vi "syncAIandAOat1MHz_v2.vi"() -> ()   [LabVIEW 2015]
uses:
  <vilib>/DAQmx/write.llb/DAQmx Write (Analog 1D Wfm NChan NSamp).vi
  <vilib>/DAQmx/read.llb/DAQmx Read (Analog 2D I16 NChan NSamp).vi
  <vilib>/DAQmx/write.llb/DAQmx Write (Analog 2D DBL NChan NSamp).vi
  <vilib>/Waveform/DWDTOps.llb/DWDT Analog to Digital.vi
  <vilib>/DAQmx/create/channels.llb/DAQmx Create Channel (AO-Voltage-Basic).vi
  <vilib>/DAQmx/create/channels.llb/DAQmx Create Channel (AI-Voltage-Basic).vi
  <vilib>/DAQmx/configure/timing.llb/DAQmx Timing (Sample Clock).vi
  <vilib>/DAQmx/miscellaneous.llb/DAQmx Fill In Error Info.vi
  <vilib>/DAQmx/configure/trigger.llb/DAQmx Start Trigger (Digital Edge).vi
  <resource>/objmgr/daqmx.rc
panel:
  in  "index (page)":i32
  out "XY Graph":T1(graph)
  in  "V":dbl=2.0 format="%#_13g"
  in  "AOrate":dbl=400000.0 format="%#_13g"
  in  "stop":bool
  out "Intensity Graph":sgl[][](graph)
  in  "error in 2":errorcluster caption="error in"
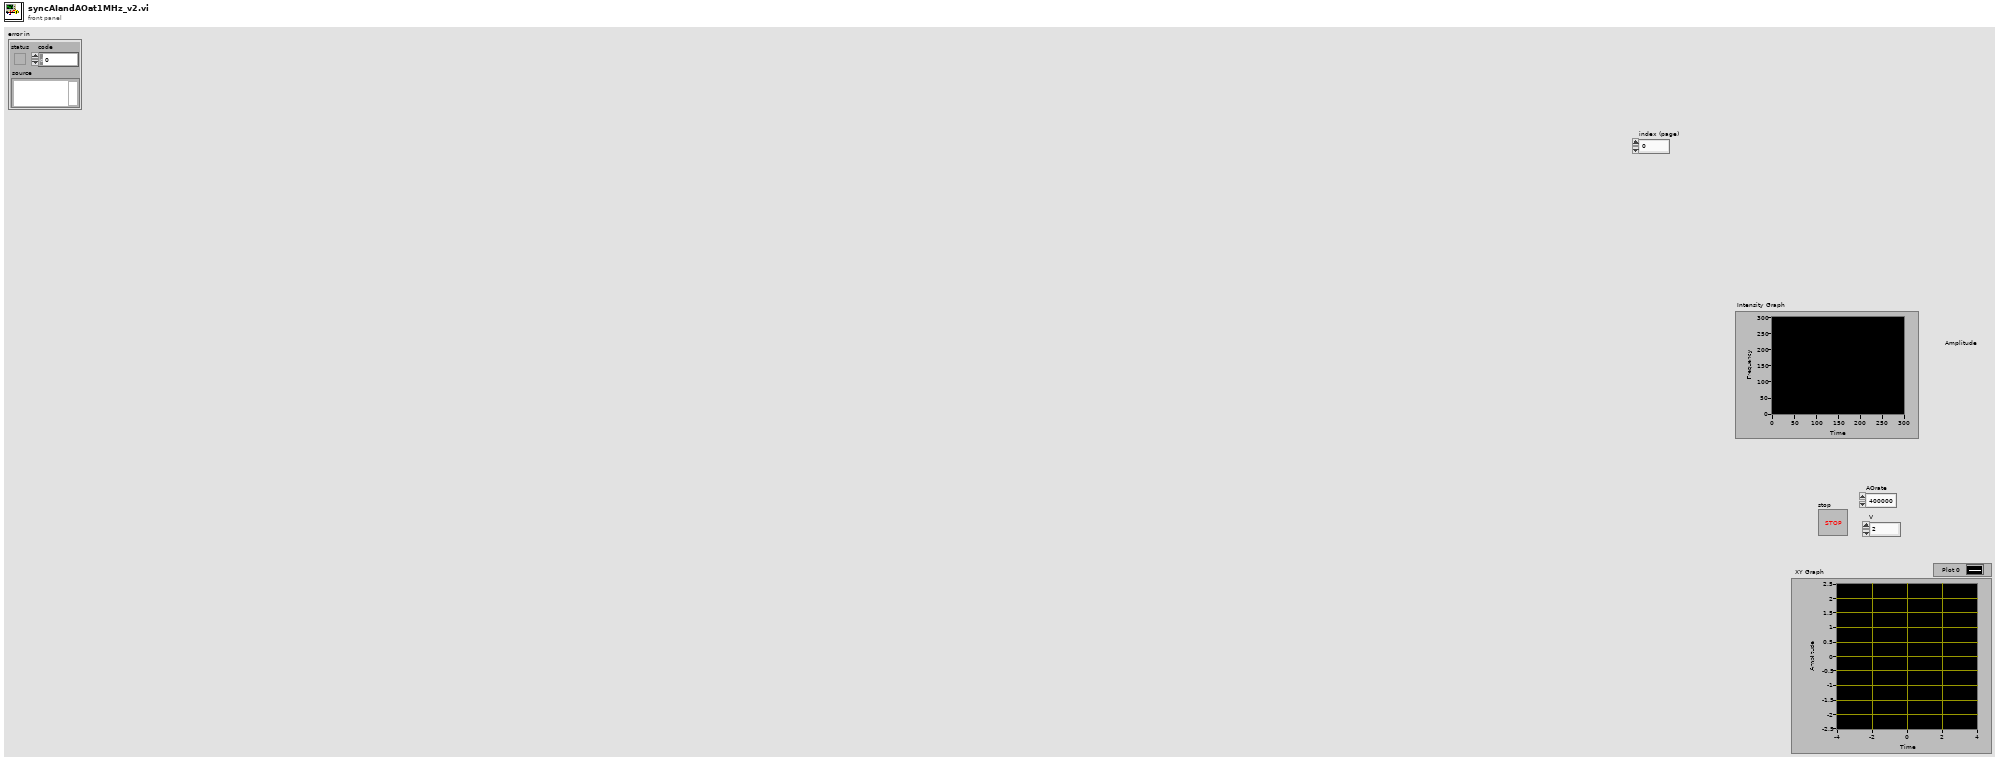
[diagram p1: front panel]
types:
  T1 = cluster{"X-WaveArray":dbl[], "Y-WaveArray":dbl[]}
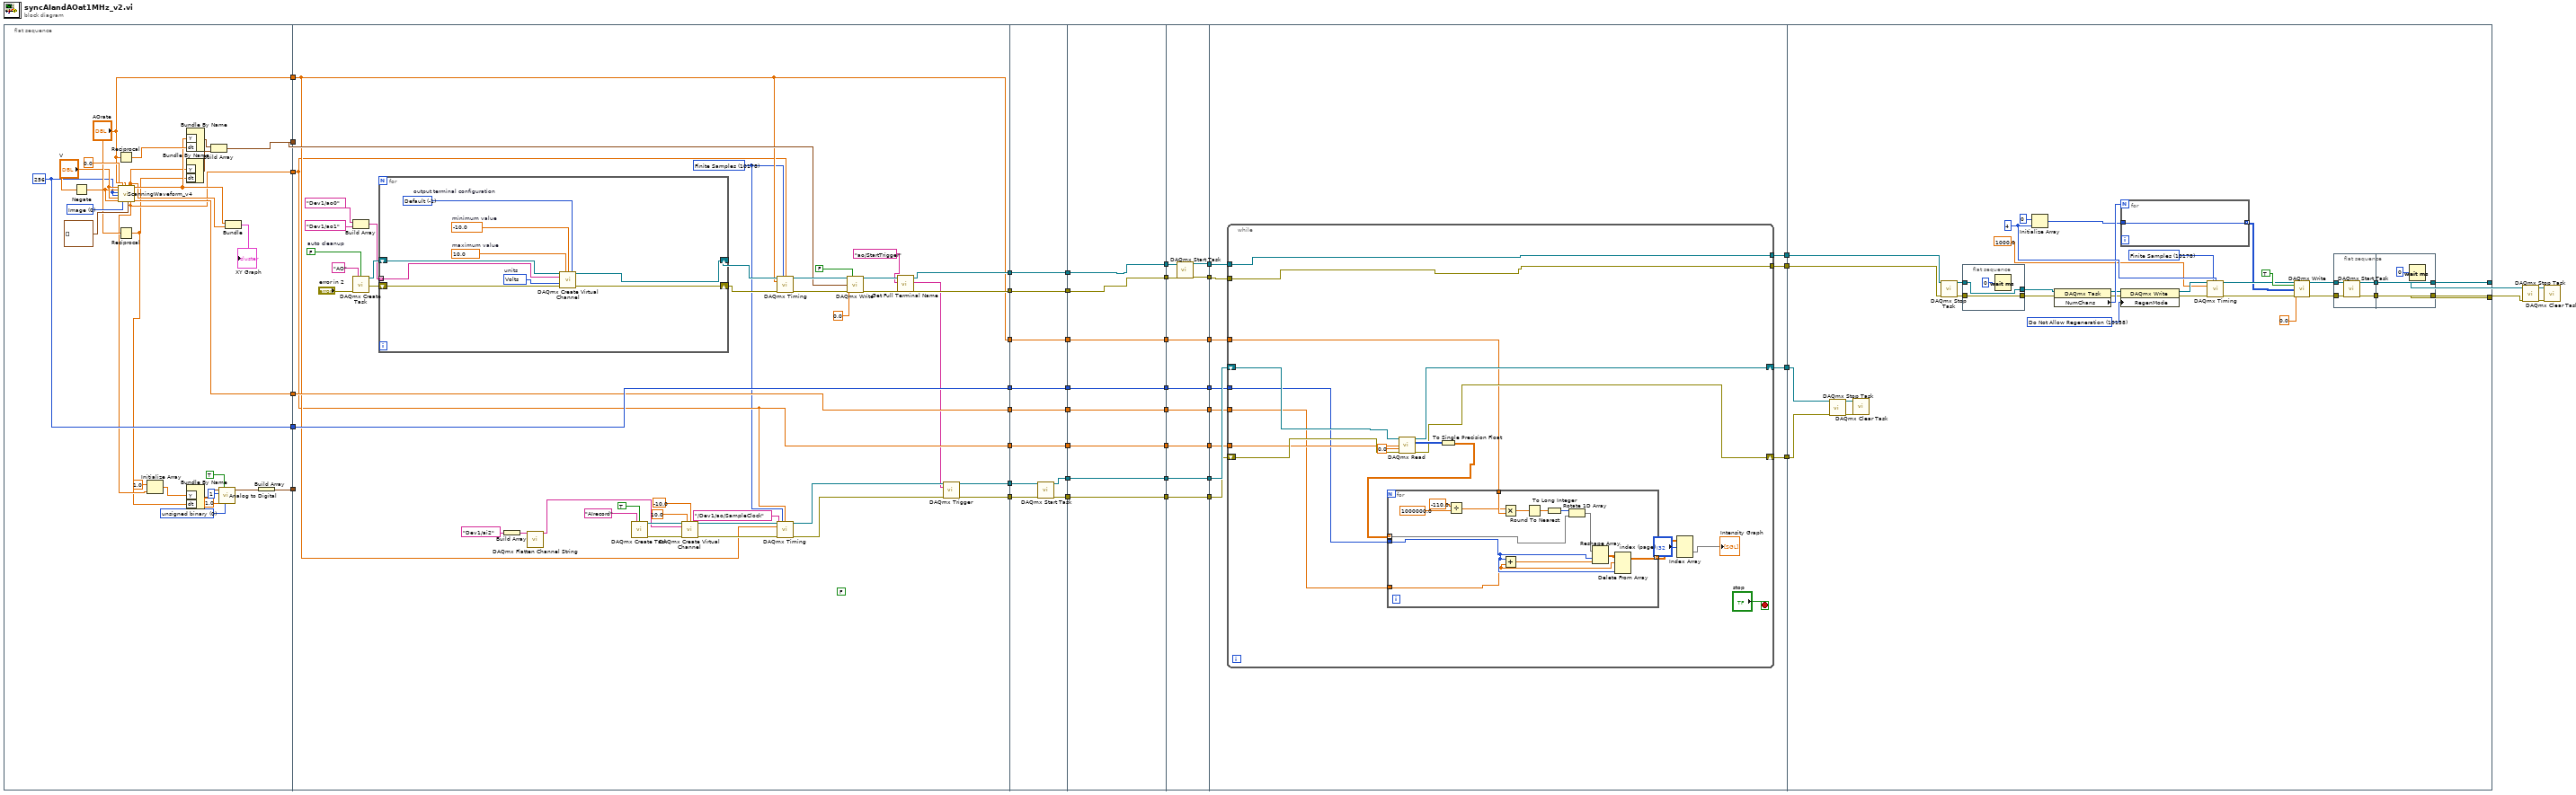
[diagram p0: block diagram]
diagram:
  n1 = flat-sequence {
    tunnel: [w61] -> w46
    tunnel: [w57] -> w45
    tunnel: ["AOrate"] -> w44
    tunnel: [w63] -> w20
    tunnel: [w62] -> w15
    tunnel: [w47] -> w7
    tunnel: w46 -> [w101]
    tunnel: w45 -> [w76]
    tunnel: w44 -> [w77]
    tunnel: [w83] -> w43
    tunnel: [w89] -> w40
    tunnel: [w87] -> w39
    tunnel: [w76] -> w25
    tunnel: [w77] -> w21
    tunnel: w20 -> [w91]
    tunnel: [w91] -> w16
    tunnel: w15 -> [w90]
    tunnel: [w90] -> w11
    tunnel: [w82] -> w10
    tunnel: w7 -> [_]
    tunnel: w43 -> [w133]
    tunnel: [w133] -> w42
    tunnel: [w132] -> w41
    tunnel: w40 -> [w131]
    tunnel: w39 -> [w130]
    tunnel: [w129] -> w33
    tunnel: [w128] -> w31
    tunnel: [w127] -> w26
    tunnel: w25 -> [w127]
    tunnel: [w126] -> w22
    tunnel: w21 -> [w126]
    tunnel: [w125] -> w17
    tunnel: w16 -> [w125]
    tunnel: [w124] -> w12
    tunnel: w11 -> [w124]
    tunnel: w10 -> [w132]
    tunnel: w42 -> [w135]
    tunnel: w41 -> [w134]
    tunnel: [w135] -> w38
    tunnel: [w134] -> w36
    tunnel: [w141] -> w34
    tunnel: w33 -> [w141]
    tunnel: [w140] -> w32
    tunnel: w31 -> [w140]
    tunnel: [w139] -> w27
    tunnel: w26 -> [w139]
    tunnel: [w138] -> w23
    tunnel: w22 -> [w138]
    tunnel: [w137] -> w18
    tunnel: w17 -> [w137]
    tunnel: [w136] -> w13
    tunnel: w12 -> [w136]
    tunnel: w38 -> [w145]
    tunnel: [w143] -> w37
    tunnel: w36 -> [w144]
    tunnel: [w142] -> w35
    tunnel: w34 -> [w151]
    tunnel: w32 -> [w150]
    tunnel: [w151] -> w30
    tunnel: [w150] -> w29
    tunnel: [w149] -> w28
    tunnel: w27 -> [w149]
    tunnel: [w148] -> w24
    tunnel: w23 -> [w148]
    tunnel: [w147] -> w19
    tunnel: w18 -> [w147]
    tunnel: [w146] -> w14
    tunnel: w13 -> [w146]
    tunnel: w37 -> [w154]
    tunnel: w35 -> [w155]
    tunnel: w30 -> [w163]
    tunnel: w29 -> [w162]
    tunnel: w28 -> [w161]
    tunnel: w24 -> [w158]
    tunnel: w19 -> [w157]
    tunnel: w14 -> [w156]
    tunnel: [w160] -> w4
    tunnel: [w159] -> w3
    tunnel: [w153] -> w2
    tunnel: [w152] -> w1
    tunnel: [w204] -> w6
    tunnel: [w203] -> w5
    tunnel: w1 -> [w205]
    tunnel: w2 -> [w206]
    tunnel: w3 -> [w199]
    tunnel: w4 -> [w200]
    frame #0 {
      w49 = u16 0 items=["unsigned binary", "offset binary", "2's complement"] ("data format (offset binary)")
      w63 = 256
      w71 = u16 0 items=["Image", "Fill Rectangle", "Fill Circle", "Draw Freeform", "Fill Freeform", "Ellipse Boundary", "Line"] ("Drawing Mode")
      n2 = Negate(x="V") -> (-x=w64:dbl)
      n3 = Reciprocal(x="AOrate") -> (1/x=w69:dbl)
      n4 = Reciprocal(x="AOrate") -> (1/x=w54:dbl)
      n5 = call "ScanningWaveform_v4.vi"("Vy-min"=w64, "Vy-max"="V", "yPixels/tPixels"=w63, "xPixels/rPixels"=w63, "Vx-min"=w64, "Vx-max"="V", "Drawing Mode"=w71, "Angle"=0.0, "AOrate"="AOrate", "Points"=cluster{"X":dbl, "Y":dbl}[] []) -> ("numPixels"=w57:dbl, "Y-WaveArray"=w59:dbl[], "P"=w62:dbl, "X-WaveArray"=w60:dbl[])  [unwired: 6 in]
      n6 = Initialize Array(1.0 ("element"), w57) -> (w55:dbl[])
      n7 = Bundle By Name("Y"=w59, "dt"=w54) -> (w67:waveform(dbl))  [unwired: 1 in]
      n8 = Bundle By Name("Y"=w60, "dt"=w69) -> (w68:waveform(dbl))  [unwired: 1 in]
      n9 = Bundle By Name("Y"=w55, "dt"=w54) -> (w53:waveform(dbl))  [unwired: 1 in]
      n10 = Build Array(w68, w67) -> (w61:waveform(dbl)[])
      n11 = call-poly <vilib>:"Analog to Digital.vi"("data format (offset binary)"=w49, "compress digital (T)"=TRUE, "full-scale range (pk-pk)"=1.0, "resolution (16 bit)"=1, "analog waveform"=w53) -> ("digital waveform"=w48:digitalwaveform)  [unwired: 3 in, 3 out]
      n12 = Bundle("X-WaveArray"=w60, "Y-WaveArray"=w59) -> (→"XY Graph":T1)  [unwired: 1 in]
      n13 = Build Array(w48) -> (w47:digitalwaveform[])
    }
    frame #1 {
      (unwired) FALSE ("auto start")
      w75 = 10178 items=["Finite Samples"=10178, "Continuous Samples"=10123, "Hardware Timed Single Point"=12522] ("sample mode")
      w112 = FALSE  # auto cleanup
      n14 = Build Array(tag "Dev1/ao0" ("physical channels"), tag "Dev1/ao1" ("physical channels")) -> (w102:tag[])
      n15 = call <vilib>:"DAQmx Create Task.vi"("new task name"="AO", "auto cleanup"=w112, "error in"="error in 2") -> ("task out"=w113:refnum<k21>, "error out"=w114:errorcluster)  [unwired: 11 in]
      n16 = for {
        shift-right: [w116] -> w109
        shift-left: w113 -> [w119]
        shift-right: [w115] -> w108
        shift-left: w114 -> [w118]
        tunnel: w102 -> [w117] mode=indexing
        w123 = -1 items=["Default"=-1, "RSE"=10083, "Differential"=10106, "Pseudodifferential"=12529]  # output terminal configuration
        w122 = 10348 items=["Volts"=10348, "From Custom Scale"=10065]  # units
        w121 = -10.0  # minimum value
        w120 = 10.0  # maximum value
        n17 = call-poly <vilib>:"DAQmx Create Virtual Channel.vi"("task in"=w119, "maximum value"=w120, "minimum value"=w121, "output terminal configuration"=w123, "physical channels"=w117, "units"=w122, "error in"=w118) -> ("task out"=w116:refnum<k21>, "error out"=w115:errorcluster)  [unwired: 7 in]
      }
      n18 = Build Array(tag "Dev1/ai2" ("physical channels")) -> (w80:tag[])
      n19 = call <vilib>:"DAQmx Flatten Channel String.vi"("names in"=w80) -> ("names out"=w78:string)  [unwired: 13 in, 1 out]
      n20 = call <vilib>:"DAQmx Create Task.vi"("new task name"="AIrecord", "auto cleanup"=TRUE) -> ("task out"=w94:refnum<k21>, "error out"=w95:errorcluster)  [unwired: 12 in]
      n21 = call-poly <vilib>:"DAQmx Create Virtual Channel.vi"("task in"=w94, "maximum value"=10.0, "minimum value"=-10.0, "physical channels"=w78, "error in"=w95) -> ("task out"=w100:refnum<k21>, "error out"=w99:errorcluster)  [unwired: 9 in]
      n22 = call-poly <vilib>:"DAQmx Timing.vi"("task/channels in"=w100, "sample mode"=w75, "samples per channel"=w76, "rate"=w77, "source"=tag "/Dev1/ao/SampleClock", "error in"=w99) -> ("task out"=w92:refnum<k21>, "error out"=w88:errorcluster)  [unwired: 8 in]
      n23 = call-poly <vilib>:"DAQmx Timing.vi"("task/channels in"=w109, "sample mode"=w75, "samples per channel"=w76, "rate"=w77, "error in"=w108) -> ("task out"=w107:refnum<k21>, "error out"=w106:errorcluster)  [unwired: 2 in, 7 out]
      n24 = call-poly <vilib>:"DAQmx Write.vi"("task/channels in"=w107, "auto start"=FALSE, "data"=w101, "timeout"=0.0, "error in"=w106) -> ("task out"=w86:refnum<k21>, "error out"=w85:errorcluster)  [unwired: 8 in, 1 out]
      n25 = call "Get Full Terminal Name.vi"("error in"=w85, "Local Terminal Name"="ao/StartTrigger", "task/channels in"=w86) -> ("error out"=w82:errorcluster, "Terminal Name with Device Prefix"=w74:tag, "task out"=w83:refnum<k21>)  [unwired: 6 in]
      n26 = call-poly <vilib>:"DAQmx Trigger.vi"("task/channels in"=w92, "source"=w74, "error in"=w88) -> ("task out"=w89:refnum<k21>, "error out"=w87:errorcluster)  [unwired: 11 in]
    }
    frame #2 {
      n27 = call <vilib>:"DAQmx Start Task.vi"("task/channels in"=w131, "error in"=w130) -> ("task out"=w129:refnum<k21>, "error out"=w128:errorcluster)  [unwired: 12 in]
    }
    frame #3 {
    }
    frame #4 {
      n28 = call <vilib>:"DAQmx Start Task.vi"("task/channels in"=w145, "error in"=w144) -> ("task out"=w143:refnum<k21>, "error out"=w142:errorcluster)  [unwired: 12 in]
    }
    frame #5 {
      n29 = while {
        tunnel: w161 -> [w177]
        tunnel: w158 -> [w172]
        tunnel: w157 -> [w171]
        tunnel: w156 -> [w170]
        shift-right: [w175] -> w160
        shift-left: w163 -> [w179]
        shift-right: [w174] -> w159
        shift-left: w162 -> [w178]
        tunnel: w155 -> [w167]
        tunnel: w154 -> [w168]
        tunnel: [w168] -> w153
        tunnel: [w167] -> w152
        stop <- "stop" stop-if-true
        n30 = call-poly <vilib>:"DAQmx Read.vi"("task/channels in"=w179, "number of samples per channel"=w177, "timeout"=0.0, "error in"=w178) -> ("task out"=w175:refnum<k21>, "data"=w180:i16[][], "error out"=w174:errorcluster)  [unwired: 9 in]
        n31 = To Single Precision Float(number=w180) -> (single precision float=w173:sgl[][])
        n32 = for {
          tunnel: w173 -> [w194] mode=indexing
          tunnel: w172 -> [w193]
          tunnel: w171 -> [w192]
          tunnel: w170 -> [w191]
          tunnel: [w181] -> w166 mode=indexing
          n33 = Divide(x=-110.0, y=1000000.0) -> (x/y=w187:dbl)
          n34 = Multiply(x=w187, y=w193) -> (x*y=w183:dbl)
          n35 = Add(x=w192, y=w191) -> (x+y=w182:dbl)
          n36 = Round To Nearest(number=w183) -> (nearest integer value=w186:dbl)
          n37 = To Long Integer(number=w186) -> (32bit integer=w184:i32)
          n38 = Rotate 1D Array(1:w194, 2:w184) -> (0:w185:sgl[])
          n39 = Reshape Array(w185, w192, w182) -> (w190:sgl[][])
          n40 = Delete From Array(array=w190, length=w191, index (col)=w192) -> (array with subset deleted=w181:sgl[][])  [unwired: 1 in, 1 out]
        }
        n41 = Index Array(array=w166, index (dim 0)="index (page)") -> (element=→"Intensity Graph":sgl[][])  [unwired: 2 in]
      }
    }
    frame #6 {
      w224 = 4 ("samples per channel")
      w210 = 10178 items=["Finite Samples"=10178, "Continuous Samples"=10123, "Hardware Timed Single Point"=12522] ("sample mode")
      w207 = 10158 items=["Allow Regeneration"=10097, "Do Not Allow Regeneration"=10158] ("RegenMode")
      n42 = call <vilib>:"DAQmx Stop Task.vi"("task/channels in"=w200, "error in"=w199) -> ("task out"=w201:refnum<k21>, "error out"=w202:errorcluster)  [unwired: 12 in]
      n43 = call <vilib>:"DAQmx Clear Task.vi"("task in"=w201, "error in"=w202) -> ()  [unwired: 13 in, 1 out]
      n44 = call <vilib>:"DAQmx Stop Task.vi"("task/channels in"=w206, "error in"=w205) -> ("task out"=w215:refnum<k21>, "error out"=w216:errorcluster)  [unwired: 12 in]
      n45 = flat-sequence {
        tunnel: w215 -> [w230]
        tunnel: [w230] -> w217
        tunnel: w216 -> [w229]
        tunnel: [w229] -> w221
        frame #0 {
          n46 = Wait (ms)(milliseconds to wait=u32 0) -> ()  [unwired: 1 out]
        }
      }
      n47 = Initialize Array(u32 0 ("element"), w224) -> (w197:u32[])
      n48 = property class="DAQmx Task"(reference=w217, error in=w221) -> (reference out=w220:refnum<k21>, error out=w222:errorcluster, "NumChans"=w223:u32)
      n49 = for {
        N: w223 -> [_]
        tunnel: w197 -> [w227]
        tunnel: [w227] -> w196 mode=indexing
      }
      n50 = property class="DAQmx Write"(reference=w220, error in=w222, "RegenMode"=w207) -> (reference out=w208:refnum<k21>, error out=w209:errorcluster)
      n51 = call-poly <vilib>:"DAQmx Timing.vi"("task/channels in"=w208, "sample mode"=w210, "samples per channel"=w224, "rate"=1000.0, "error in"=w209) -> ("task out"=w211:refnum<k21>, "error out"=w212:errorcluster)  [unwired: 9 in]
      n52 = call-poly <vilib>:"DAQmx Write.vi"("task/channels in"=w211, "auto start"=TRUE, "data"=w196, "timeout"=0.0, "error in"=w212) -> ("task out"=w213:refnum<k21>, "error out"=w214:errorcluster)  [unwired: 8 in, 1 out]
      n53 = flat-sequence {
        tunnel: [w232] -> w226
        tunnel: [w231] -> w225
        tunnel: w213 -> [w234]
        tunnel: w214 -> [w233]
        tunnel: [w236] -> w203
        tunnel: [w237] -> w204
        tunnel: w226 -> [w237]
        tunnel: w225 -> [w236]
        frame #0 {
          n54 = call <vilib>:"DAQmx Start Task.vi"("task/channels in"=w234, "error in"=w233) -> ("task out"=w232:refnum<k21>, "error out"=w231:errorcluster)  [unwired: 12 in]
        }
        frame #1 {
          n55 = Wait (ms)(milliseconds to wait=u32 0) -> ()  [unwired: 1 out]
        }
      }
    }
  }
  n56 = call <vilib>:"DAQmx Stop Task.vi"("task/channels in"=w6, "error in"=w5) -> ("task out"=w9:refnum<k21>, "error out"=w8:errorcluster)  [unwired: 12 in]
  n57 = call <vilib>:"DAQmx Clear Task.vi"("task in"=w9, "error in"=w8) -> ()  [unwired: 13 in, 1 out]
